vi "Robot Global Data.vi"() -> ()   [LabVIEW 2017]
doc: "This global VI can contain as many global variables as you need. Place a control on the panel, give it a good name. To read or write to it from a VI, drag the icon to the diagram of that VI. You can also drag from the project. Click on the node to change which global you access. You shouldn't have multiple locations writing to a global or it will cause a race-condition."
uses:
  <vilib>/Rock Robotics/WPI/Camera/WPI_CameraImageSize.ctl
  <vilib>/Rock Robotics/WPI/DriverStation/WPI_DriverStationRobotMode2.ctl
panel:
  in  "LL step 4":dbl
  in  "LL step 3":dbl
  in  "wrist degrees/s":dbl
  in  "lift in/s":dbl
  in  "LL Step 2":dbl
  in  "drive train in/s":dbl
  in  "LL Step 1":dbl
  in  "Array Step":dbl
  in  "Wrist Reset":bool
  in  "Lift Reset":bool
  in  "Low gear - high gear":bool
  in  "Wrist Angle":dbl
  in  "Lift Distance":dbl
  in  "Right Rate Percent":dbl
  in  "Left Rate Percent":dbl
  in  "Right Reset":bool
  in  "Left Reset":bool
  in  "Right Rate":dbl
  in  "Right Distance":dbl
  in  "Left Rate":dbl
  in  "Left Distance":dbl
  in  "Robot Mode":T1
  in  "image size":T2=enum."320x240"
  in  "Enable Vision":bool
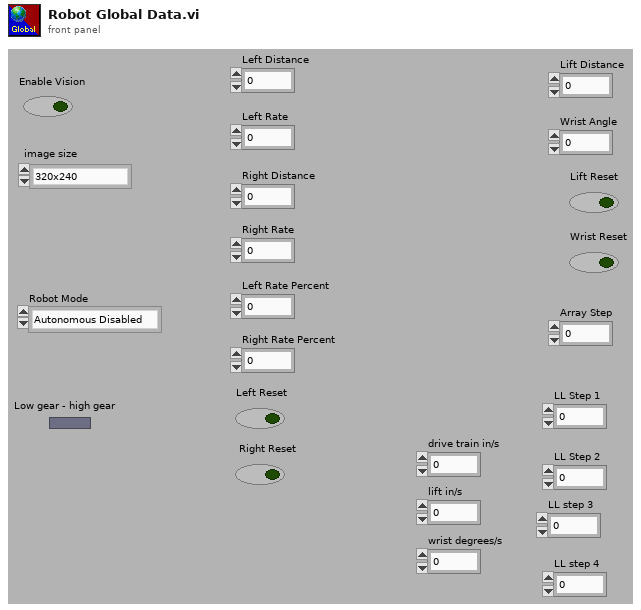
[diagram p1: front panel]
types:
  T1 = typedef "WPI_DriverStationRobotMode2.ctl" = enum16{"Autonomous Disabled", "Autonomous Enabled", "Teleop Disabled", "Teleop Enabled", "Disconnected", "Finish", "Test Disabled", "Test Enabled", "Emergency Stopped"}
  T2 = typedef "WPI_CameraImageSize.ctl" = enum16{"640x480", "320x240", "160x120", "Custom"}
diagram:
